vi "Get Node Type from Tag Name.vi"(11 "Tag Name":string) -> (1 "Type Found?":bool, 3 "Node Type":string)   [LabVIEW 2025]
uses:
  <vilib>/regexp/Match Regular Expression.xnode
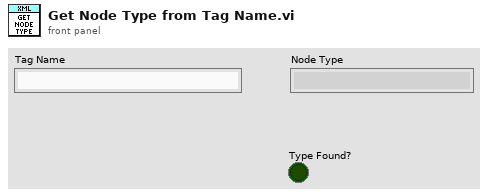
[diagram p1: front panel]
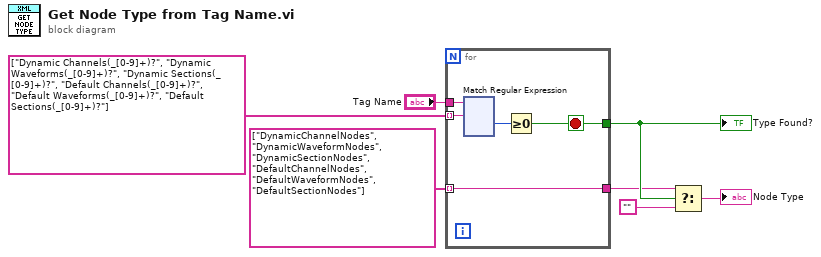
[diagram p0: block diagram]
diagram:
  n1 = for {
    tunnel: string[] ["Dynamic Channels(_[0-9]+)?", "Dynamic Waveforms(_[0-9]+)?", "Dynamic Sections(_[0-9]+)?", "Default Channels(_[0-9]+)?", "Default Waveforms(_[0-9]+)?", "Default Sections(_[0-9]+)?"] -> [w12] mode=indexing
    tunnel: "Tag Name" -> [w11]
    tunnel: string[] ["DynamicChannelNodes", "DynamicWaveformNodes", "DynamicSectionNodes", "DefaultChannelNodes", "DefaultWaveformNodes", "DefaultSectionNodes"] -> [w9] mode=indexing
    tunnel: [w9] -> w1
    tunnel: [w8] -> w4
    stop <- w8 stop-if-true
    n2 = xnode "Match Regular Expression"("input string"=w11, "regular expression"=w12) -> ("offset past match"=w10:i32)  [unwired: 4 in, 4 out]
    n3 = Greater Or Equal To 0?(x=w10) -> (x >= 0?=w8:bool)
  }
  "Type Found?" <- w4
  n4 = Select(t=w1, s=w4, f="") -> (s? t:f=→"Node Type":string)
